vi "Get PID.vi"(8 "error in":errorcluster, 11 "TE Cooler in":refnum<class "TE Cooler.lvclass">) -> (0 "error out":errorcluster, 2 "PID":cluster{"P":sgl, "I":sgl, "D":sgl}, 3 "TE Cooler out":refnum<class "TE Cooler.lvclass">)   [LabVIEW 2015, in "TE Cooler.lvlib" / "TE Cooler.lvclass"]
uses:
  TE Cooler.lvclass
  Controls/Command.ctl
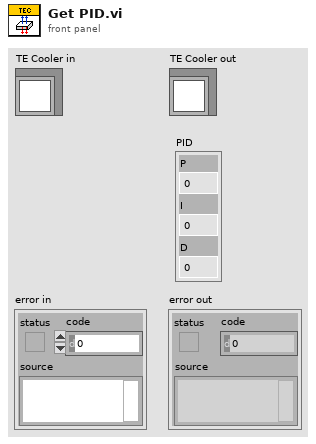
[diagram p1: front panel]
types:
  T1 = typedef "TE Cooler.lvlib/TE Cooler.lvclass/Command.ctl" = enum16{"INPUT1", "DESIRED CONTROL VALUE", "POWER OUTPUT", "ALARM STATUS", "INPUT 2", "OUTPUT CURRENT COUNTS", "ALARM TYPE", "SET TYPE DEFINE", "SENSOR TYPE", "CONTROL TYPE", "CONTROL OUTPUT POLARITY", "POWER ON/OFF", "OUTPUT SHUTDOWN IF ALARM", "FIXED DESIRED CONTROL SETTING", "PROPORTIONAL BANDWIDTH", "INTEGRAL GAIN", "DERIVATIVE GAIN", "LOW EXTERNAL SET RANGE", "HIGH EXTERNAL SET RANGE", "ALARM DEADBAND", "HIGH ALARM SETTING", "LOW ALARM SETTING", "CONTROL DEADBAND SETTING", "INPUT1 OFFSET", "INPUT2 OFFSET", "HEAT MULTIPLIER", "COOL MULTIPLIER", "OVER CURRENT COUNT COMPARE VALUE", "ALARM LATCH ENABLE", "NOT USED", "ALARM LATCH RESET", "CHOOSE SENSOR FOR ALARM FUNCTION", "CHOOSE TEMPERATURE WORKING UNITS", "EEPROM WRITE ENABLE", "OVER CURRENT CONTINUOUS", "OVER CURRENT RESTART ATTEMPTS", "JP3 DISPLAY ENABLE"}
  T2 = cluster{"scaledOut":sgl, "scaledOut":sgl, "scaledOut":sgl}
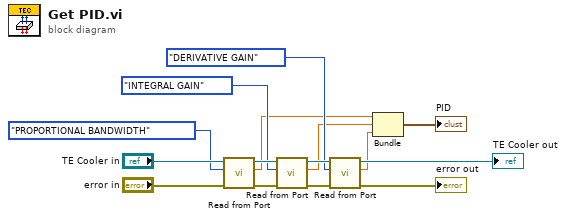
[diagram p0: block diagram]
diagram:
  n1 = call "Read from Port.vi"("error in"="error in", "TEC Cmd"=Command."PROPORTIONAL BANDWIDTH", "TE Cooler in"="TE Cooler in") -> ("error out"=w8:errorcluster, "scaledOut"=w3:sgl, "TE Cooler out"=w9:refnum<class "TE Cooler.lvclass">)  [unwired: 5 in, 1 out]
  n2 = call "Read from Port.vi"("error in"=w8, "TEC Cmd"=Command."INTEGRAL GAIN", "TE Cooler in"=w9) -> ("error out"=w5:errorcluster, "scaledOut"=w2:sgl, "TE Cooler out"=w6:refnum<class "TE Cooler.lvclass">)  [unwired: 5 in, 1 out]
  n3 = call "Read from Port.vi"("error in"=w5, "TEC Cmd"=Command."DERIVATIVE GAIN", "TE Cooler in"=w6) -> ("error out"=→"error out":errorcluster, "scaledOut"=w1:sgl, "TE Cooler out"=→"TE Cooler out":refnum<class "TE Cooler.lvclass">)  [unwired: 5 in, 1 out]
  n4 = Bundle("scaledOut"=w3, "scaledOut"=w2, "scaledOut"=w1) -> (→"PID":T2)  [unwired: 1 in]
